vi "Name_ICM_Gap.vi"() -> (3 "Name":string)   [LabVIEW 2015, in "Exposure Process.lvlib"]
uses:
  Exposure Process.lvlib
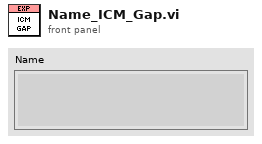
[diagram p1: front panel]
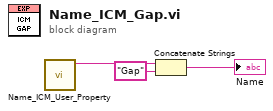
[diagram p0: block diagram]
diagram:
  n1 = call "Name_ICM_User_Property.vi"() -> ("Name"=w3:string)  [unwired: 11 in]
  n2 = Concatenate Strings(w3, "Gap" ("string")) -> (→"Name":string)
